vi "Read PWM Input Channel.vi"(8 "error in":errorcluster, 11 "PWM input channel in":refnum<class "PWM Input Channel.lvclass">) -> (0 "error out":errorcluster, 1 "measurement type":T1, 2 "default value":dbl, 3 "PWM input channel out":refnum<class "PWM Input Channel.lvclass">, 4 "index":i32, 5 "name":string)   [LabVIEW 2017, in "Scan Engine Scripting.lvlib" / "PWM Input Channel.lvclass"]
uses:
  PWM Input Channel.lvclass
  Measurement Type.ctl
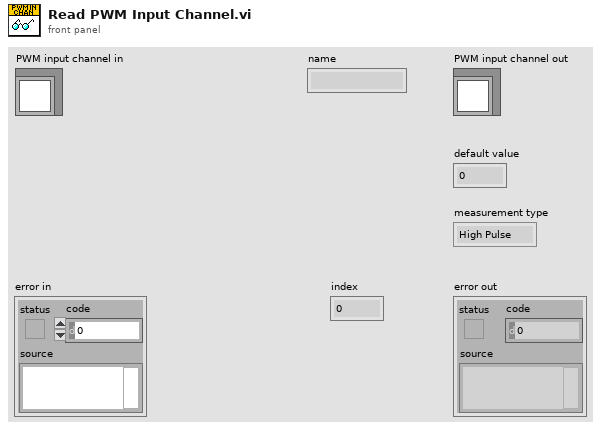
[diagram p1: front panel]
types:
  T1 = typedef "Scan Engine Scripting.lvlib/PWM Input Channel.lvclass/Measurement Type.ctl" = enum16{"High Pulse", "Low Pulse", "Most Recent"}
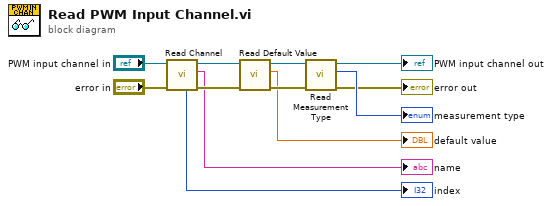
[diagram p0: block diagram]
diagram:
  n1 = call-dynamic "Read Channel.vi"("error in"="error in", "channel in"="PWM input channel in") -> ("error out"=w11:errorcluster, "name"=→"name":string, "channel out"=w9:refnum<class "PWM Input Channel.lvclass">, "index"=→"index":i32)  [unwired: 4 in, 2 out]
  n2 = call-dynamic "Read Default Value.vi"("error in"=w11, "PWM channel in"=w9) -> ("error out"=w10:errorcluster, "default value"=→"default value":dbl, "PWM channel out"=w8:refnum<class "PWM Input Channel.lvclass">)  [unwired: 7 in]
  n3 = call-dynamic "Read Measurement Type.vi"("error in"=w10, "PWM input channel in"=w8) -> ("error out"=→"error out":errorcluster, "measurement type"=→"measurement type":T1, "PWM input channel out"=→"PWM input channel out":refnum<class "PWM Input Channel.lvclass">)  [unwired: 7 in]
